vi "1D U64 To String with Interval.vi"(5 "Interval":string=",", 10 "Array In":u64[](array[numeric])) -> (2 "String out":string)   [LabVIEW 2024]
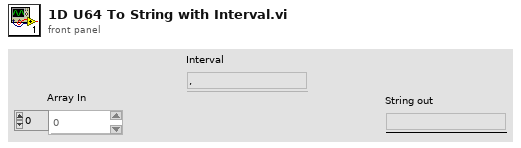
[diagram p1: front panel]
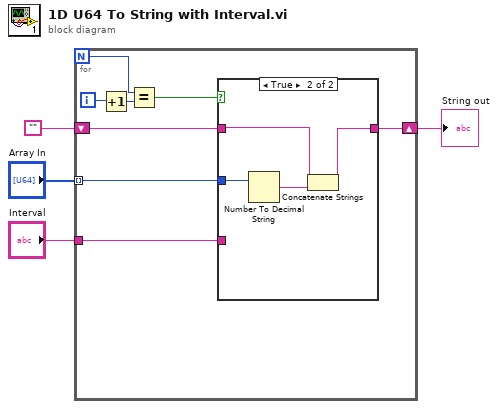
[diagram p0: block diagram]
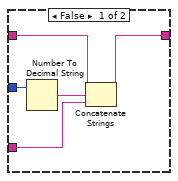
[diagram p2: hidden frame]
diagram:
  n1 = for {
    N -> [w6]
    tunnel: "Array In" -> [w12] mode=indexing
    shift-right: [w10] -> w2
    shift-left: "" -> [w11]
    tunnel: "Interval" -> [w9]
    i -> [w8]
    n2 = Increment(x=w8) -> (x+1=w7:i32)
    n3 = Equal?(x=w6, y=w7) -> (x = y?=w5:bool)
    n4 = case shown="True" w5 {
      tunnel: w12 -> [w17 w20]
      tunnel: w11 -> [w15 w19]
      tunnel: [w14 w18] -> w10
      tunnel: w9 -> [w13 _]
      frame False {
        n5 = Number To Decimal String(number=w17) -> (decimal integer string=w16:string)  [unwired: 1 in]
        n6 = Concatenate Strings(w15, w16, w13) -> (w14:string)
      }
      frame True {
        n7 = Number To Decimal String(number=w20) -> (decimal integer string=w21:string)  [unwired: 1 in]
        n8 = Concatenate Strings(w19, w21) -> (w18:string)
      }
    }
  }
  "String out" <- w2
